vi "Pa2dBSPL (SubVI).vi"(11 "Positve Half of FFT with 0Hz and Nyquist":dbl[](array[numeric])) -> (3 "dB SPL":dbl[](array[numeric]))   [LabVIEW 2015]
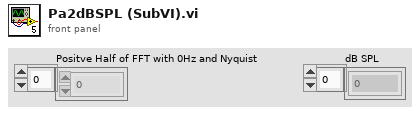
[diagram p1: front panel]
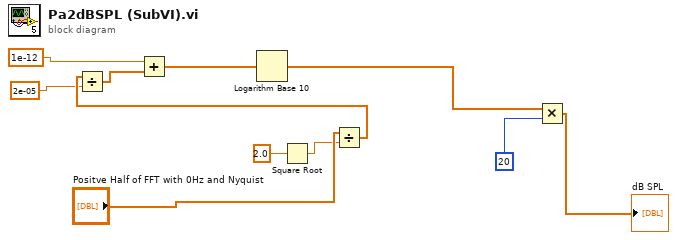
[diagram p0: block diagram]
diagram:
  n1 = Square Root(x=2.0) -> (sqrt(x)=w9:dbl)
  n2 = Divide(x="Positve Half of FFT with 0Hz and Nyquist", y=w9) -> (x/y=w11:dbl[])
  n3 = Divide(x=w11, y=2e-05) -> (x/y=w5:dbl[])
  n4 = Add(x=1e-12, y=w5) -> (x+y=w6:dbl[])
  n5 = Logarithm Base 10(1:w6) -> (0:w1:dbl[])
  n6 = Multiply(x=w1, y=20) -> (x*y=→"dB SPL":dbl[])
